vi "StepperMotorDriveDOs.vi"() -> ()   [LabVIEW 2020, in "CTI-Scratchpad.lvlib"]
uses:
  CTI-Scratchpad.lvlib
  CTI/Identity.ctl
  CTI/GPIO Direction.ctl
  CTI/GPIO Number.ctl
  CTI/Session/Session.lvclass
  CTI/CTI.lvlib
  CTI/VisaComms/VisaComms.lvclass
panel:
  in  "Speed":dbl(knob) scale=0.0..30000.0
  in  "Enable":bool
  in  "Direction":bool
  out "Numeric":i32
  out "Identity":T1
  in  "Port":refnum<visa-resource-name>="COM6"
  in  "stop":bool
  # "Could do with a soft start"
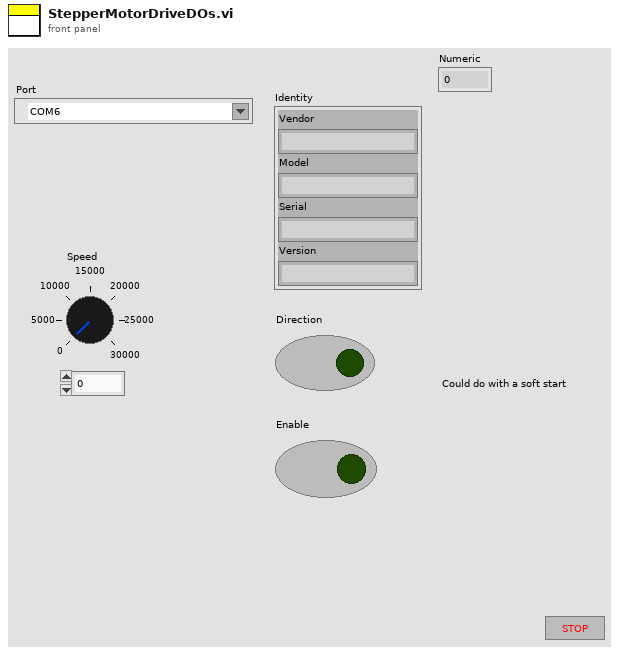
[diagram p1: front panel]
types:
  T1 = typedef "CTI.lvlib/Identity.ctl" = cluster{"Vendor":string, "Model":string, "Serial":string, "Version":string}
  T2 = typedef "CTI.lvlib/GPIO Number.ctl" = i8
  T3 = typedef "CTI.lvlib/GPIO Direction.ctl" = enum16{"In", "Out"}
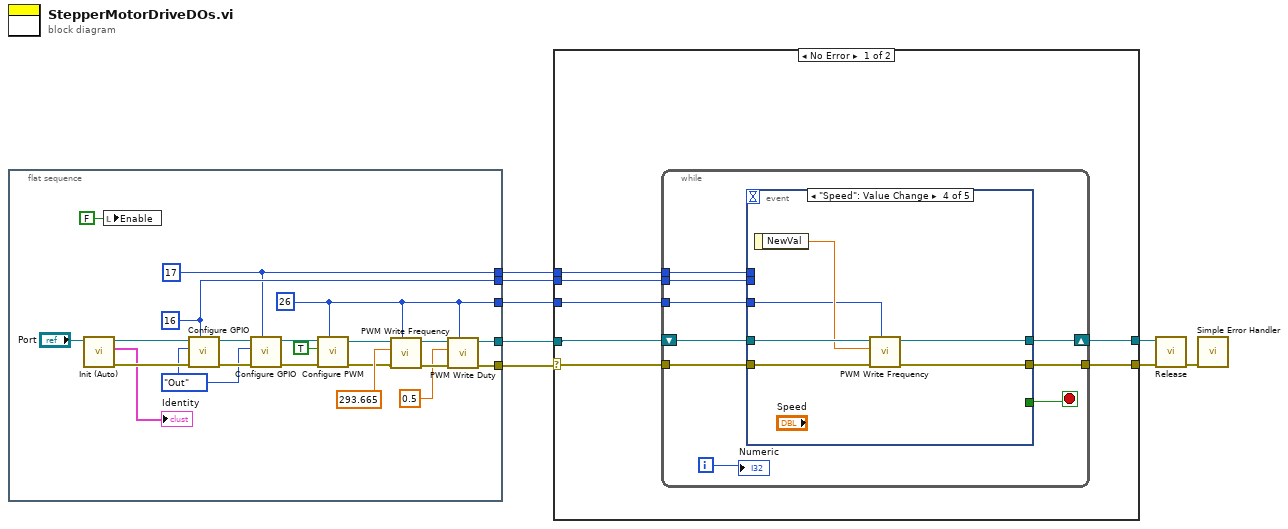
[diagram p0: block diagram]
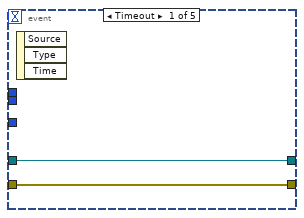
[diagram p2: hidden frame]
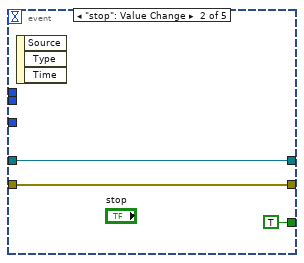
[diagram p3: hidden frame]
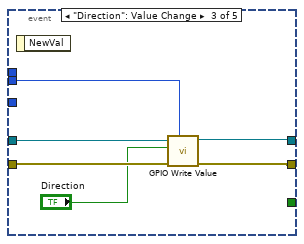
[diagram p4: hidden frame]
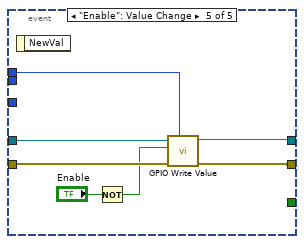
[diagram p5: hidden frame]
diagram:
  n1 = flat-sequence {
    tunnel: [w26] -> w5
    tunnel: [w23] -> w4
    tunnel: [w12] -> w3
    tunnel: [w11] -> w2
    tunnel: [w9] -> w1
    frame #0 {
      w9 = T2 26 ("GPIO #")
      w23 = T2 17 ("GPIO #")
      w26 = T2 16 ("GPIO #")
      w22 = GPIO_Direction."Out" ("GPIO Direction")
      n2 = call "Init (Auto).vi"("VISA resource name"="Port") -> ("error out"=w28:errorcluster, "Identity"=→"Identity":T1, "Session"=w29:refnum<class "Session.lvclass">)  [unwired: 8 in]
      n3 = local write "Enable"(FALSE ("Enable")) -> ()
      n4 = call "Configure GPIO.vi"("GPIO #"=w26, "error in (no error)"=w28, "GPIO Direction"=w22, "Session in"=w29) -> ("error out"=w25:errorcluster, "Session out"=w24:refnum<class "Session.lvclass">)  [unwired: 6 in]
      n5 = call "Configure GPIO.vi"("GPIO #"=w23, "error in (no error)"=w25, "GPIO Direction"=w22, "Session in"=w24) -> ("error out"=w18:errorcluster, "Session out"=w19:refnum<class "Session.lvclass">)  [unwired: 6 in]
      n6 = call "Configure PWM.vi"("GPIO #"=w9, "error in (no error)"=w18, "Enable (F)"=TRUE, "Session in"=w19) -> ("error out"=w14:errorcluster, "Session out"=w13:refnum<class "Session.lvclass">)  [unwired: 6 in]
      n7 = call "PWM Write Frequency.vi"("GPIO #"=w9, "error in (no error)"=w14, "Frequency Hz"=293.665 ("Frequency (0 Hz)"), "Session in"=w13) -> ("error out"=w17:errorcluster, "Session out"=w15:refnum<class "Session.lvclass">)  [unwired: 6 in]
      n8 = call "PWM Write Duty.vi"("GPIO #"=w9, "error in (no error)"=w17, "Duty % (0-1)"=sgl 0.5, "Session in"=w15) -> ("error out"=w11:errorcluster, "Session out"=w12:refnum<class "Session.lvclass">)  [unwired: 6 in]
    }
  }
  n9 = case shown="No Error" w2 {
    selector: w2 -> [w37 w72]
    tunnel: [w36 w71] -> w6
    tunnel: [w35 w72] -> w8
    tunnel: w5 -> [w34 _]
    tunnel: w4 -> [w33 _]
    tunnel: w3 -> [w32 w71]
    tunnel: w1 -> [w31 _]
    frame No Error {
      n10 = while {
        shift-right: [w41] -> w36
        shift-left: w32 -> [w46]
        tunnel: w34 -> [w44]
        tunnel: w33 -> [w39]
        tunnel: w37 -> [w45]
        tunnel: [w42] -> w35
        tunnel: w31 -> [w38]
        i -> [w40]
        stop <- w43 stop-if-true
        n11 = event shown="[3] \"Speed\": Value Change" {
          selector: _ -> [_ _ _ _ _]
          dyn-events: _ -> [_ _ _ _ _]
          timeout: _ -> [_ _ _ _ _]
          tunnel: w46 -> [w47 w49 w56 w63 w69]
          tunnel: w45 -> [w48 w50 w57 w62 w70]
          tunnel: w44 -> [_ _ w52 _ _]
          tunnel: [_ TRUE ("stop") _ _ _] -> w43
          tunnel: [w48 w50 w55 w60 w68] -> w42
          tunnel: [w47 w49 w54 w61 w67] -> w41
          tunnel: w39 -> [_ _ _ _ w64]
          tunnel: w38 -> [_ _ _ w58 _]
          event Timeout {
            n12 = event-data() -> ()  [unwired: 1 in, 3 out]
          }
          event "stop": Value Change {
            n13 = event-data() -> ()  [unwired: 1 in, 3 out]
          }
          event "Direction": Value Change {
            n14 = event-data() -> ()  [unwired: 1 in, 1 out]
            n15 = call "GPIO Write Value.vi"("GPIO #"=w52, "error in (no error)"=w57, "Value"="Direction", "Session in"=w56) -> ("error out"=w55:errorcluster, "Session out"=w54:refnum<class "Session.lvclass">)  [unwired: 6 in]
          }
          event "Speed": Value Change {
            n16 = event-data() -> ("NewVal"=w59:dbl)  [unwired: 1 in]
            n17 = call "PWM Write Frequency.vi"("GPIO #"=w58, "error in (no error)"=w62, "Frequency Hz"=w59, "Session in"=w63) -> ("error out"=w60:errorcluster, "Session out"=w61:refnum<class "Session.lvclass">)  [unwired: 6 in]
          }
          event "Enable": Value Change {
            n18 = event-data() -> ()  [unwired: 1 in, 1 out]
            n19 = Not(x="Enable") -> (.not. x?=w65:bool)
            n20 = call "GPIO Write Value.vi"("GPIO #"=w64, "error in (no error)"=w70, "Value"=w65, "Session in"=w69) -> ("error out"=w68:errorcluster, "Session out"=w67:refnum<class "Session.lvclass">)  [unwired: 6 in]
          }
        }
        "Numeric" <- w40
      }
    }
    frame Error {
    }
  }
  n21 = call-dynamic "Release.vi"("error in (no error)"=w8, "Session in"=w6) -> ("error out"=w7:errorcluster)  [unwired: 9 in]
  n22 = call <vilib>:"Simple Error Handler.vi"("error in (no error)"=w7) -> ()  [unwired: 4 in, 5 out]
